vi "ActorPlugin-004-SpecificationCenter.vi"(0 "FTW Actor Instance Configuration":string="{\n  \"Identity\": \"ActorName\",\n  \"InboxAddress\": \"tcp://127.0.0.1:*\",\n  \"PublisherAddress\": \"tcp://127.0.0.1:*\",\n  \"DebugEnableInboxLogging\": false,\n  \"DebugEnableJobLogging\": false,\n  \"DebugShowPanel\": false\n}", 11 "Error In":errorcluster) -> (15 "Error":errorcluster)   [LabVIEW 2013, in "ERP-SpecificationManager.lvclass"]
uses:
  Actors/ERP-Specification Center/ERP-SpecificationManager.lvclass
  Actors/ERP-Specification Center/Controls/Spec-ManageExisting.ctl
  Actors/ERP-Specification Center/Controls/Spec-CreateNew.ctl
  Actors/ERP-Specification Center/ERP-SpecificationManager.lvclass/ERP-SpecificationManager.ctl
  ftw-dataflow/Actor/src/Instance/FTW-ActorInstance.lvclass
  ftw-dataflow/Actor/src/Message/Request/FTW-Message-IncomingRequest.lvclass
  ERP-ConfigPageNewFeather/PCert-ConfigPageNF.lvclass
panel:
  in  "Spec New":T1
  in  "Spec Manager":T2
  in  "Tab Control":T3(tab)
  in  "Refresh Table":bool
  in  "Delete Part":bool
  in  "Tables":u16(ring) items=["Aluminum Oxide Items", "CCW Items", "Other Items", "Probe Clean Items", "Probe Form Items", "Probe Lap Items", "Probe Polish Items", "Probe Scrub Items"]
  in  "Udpate Description":bool
  in  "Description Updater":string
  in  "Clear Search":bool
  in  "Part Number":string
  in  "Search Button":bool
  in  "Specification Table":string[][](table)
  # "Specification Controls"
  # "Welcome to the ITS Specification Manager\nPlease use the Controls below to \naccess the system."
  # "Update Part Number Description Option"
  # "Search Controls"
  # "Table Selection"
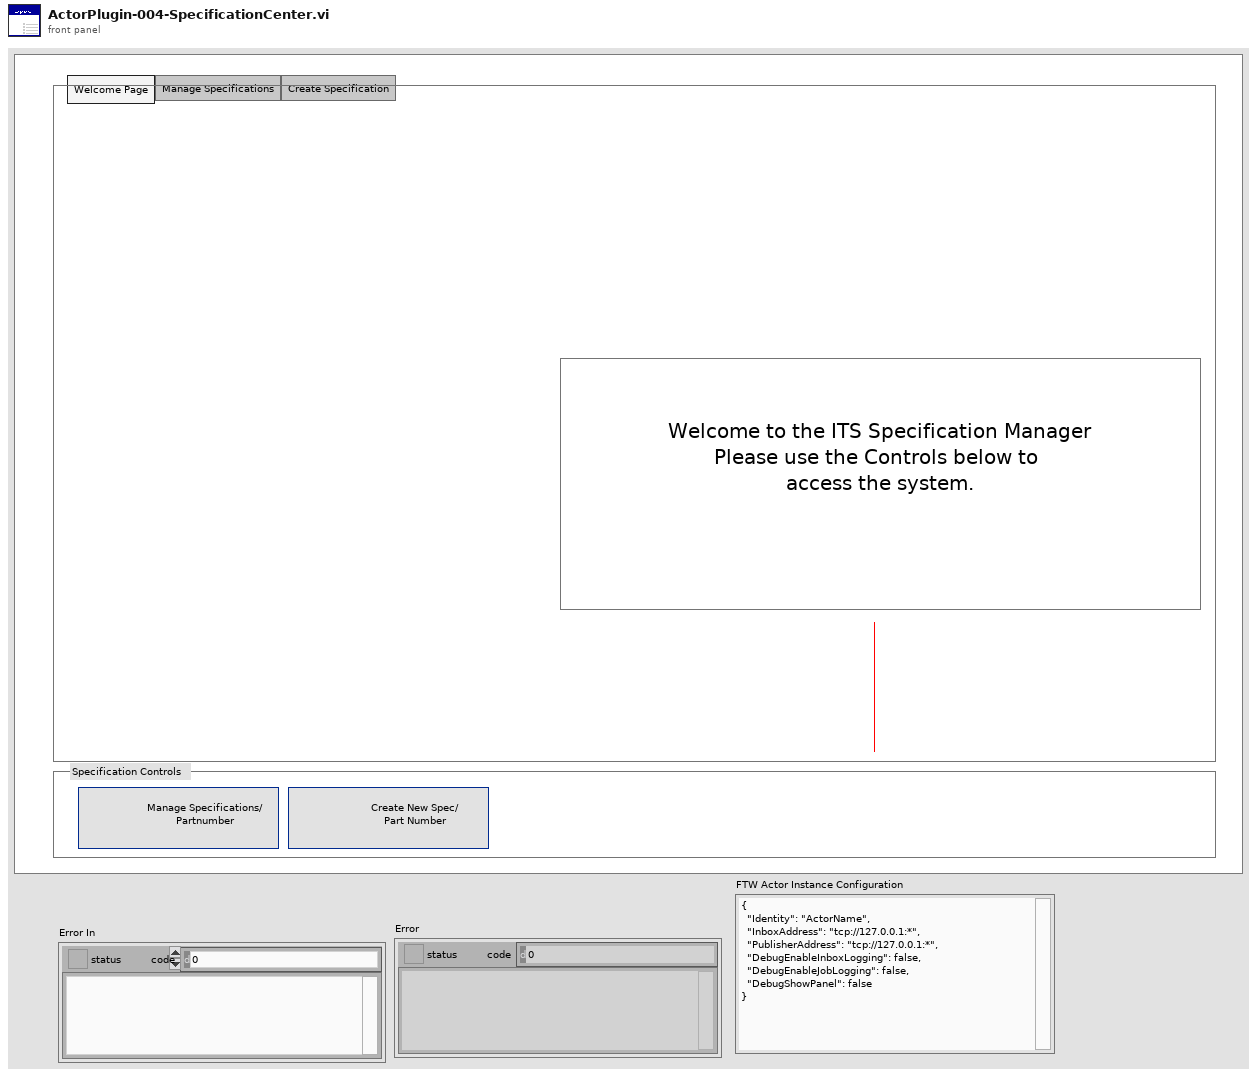
[diagram p1: front panel]
types:
  T1 = typedef "ERP-SpecificationManager.lvclass/Spec-CreateNew.ctl" = bool
  T2 = typedef "ERP-SpecificationManager.lvclass/Spec-ManageExisting.ctl" = bool
  T3 = enum32{"Welcome Page", "Manage Specifications", "Create Specification"}
  T4 = cluster{"Incoming Requests":refnum<event-registration>}
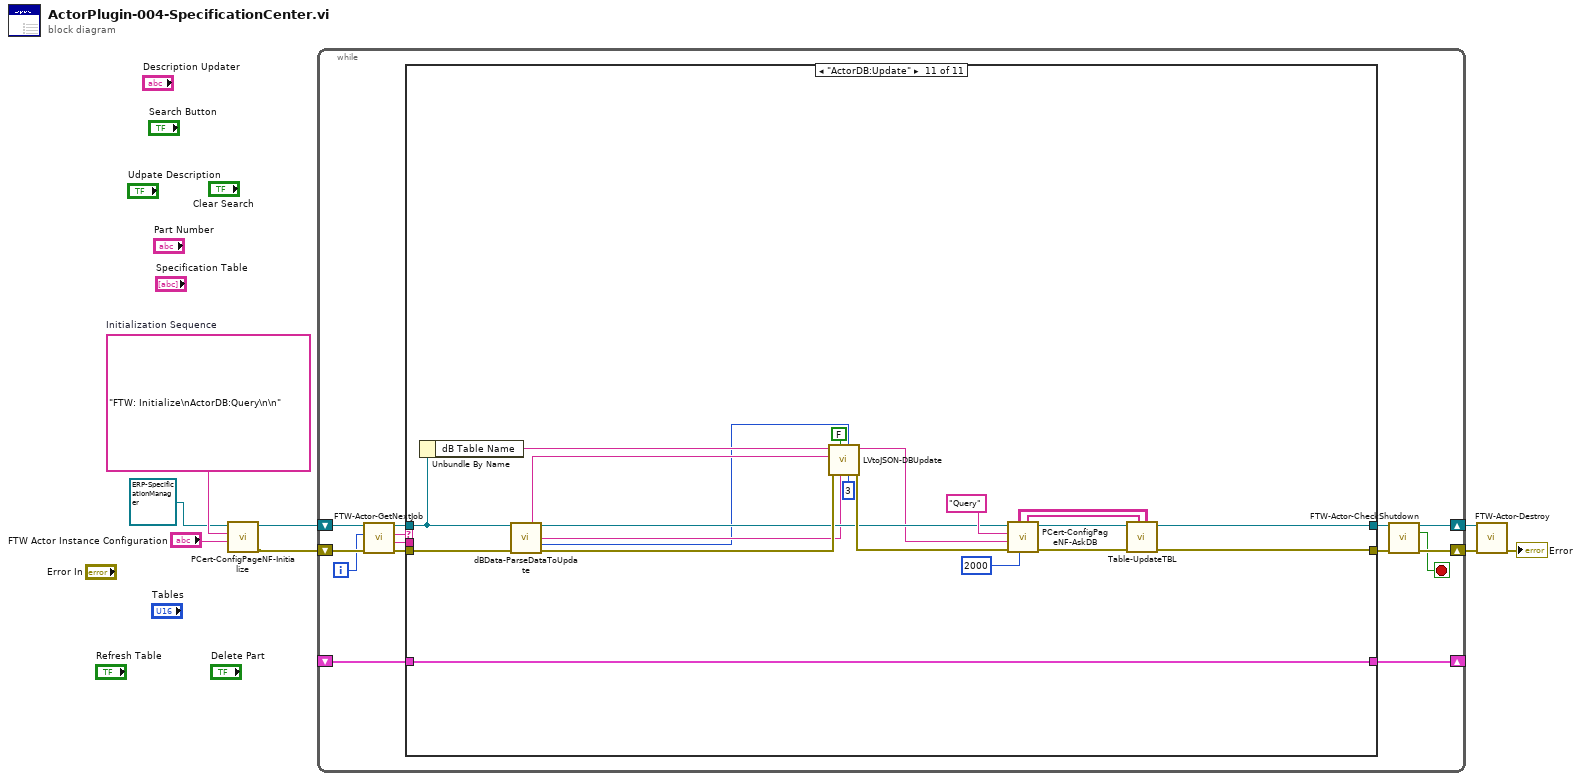
[diagram p0: block diagram]
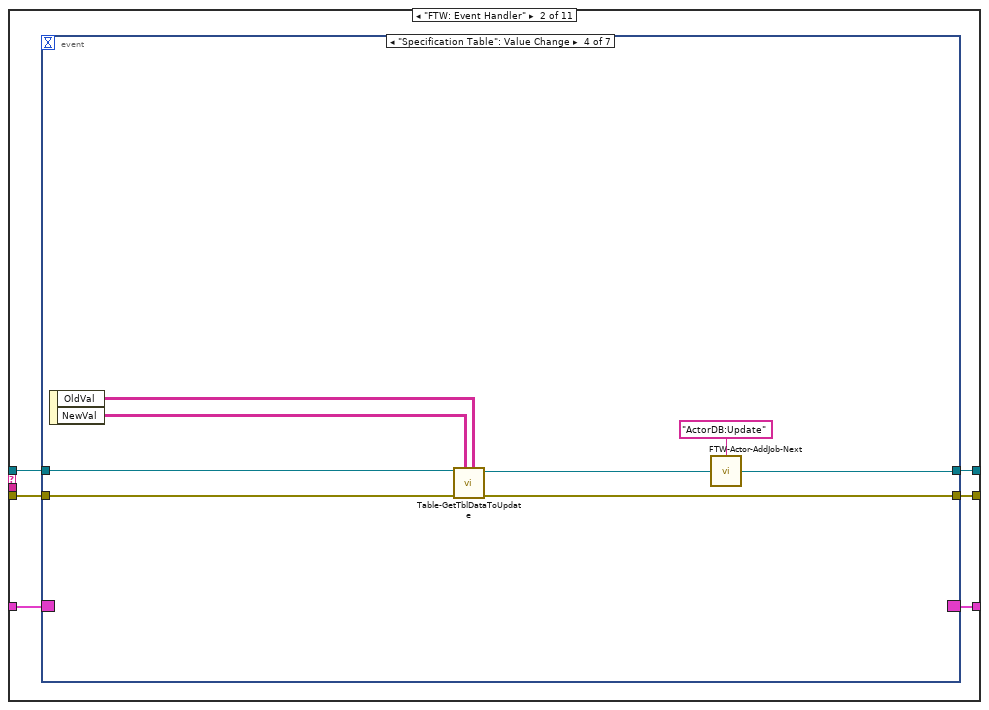
[diagram p3: hidden frame]
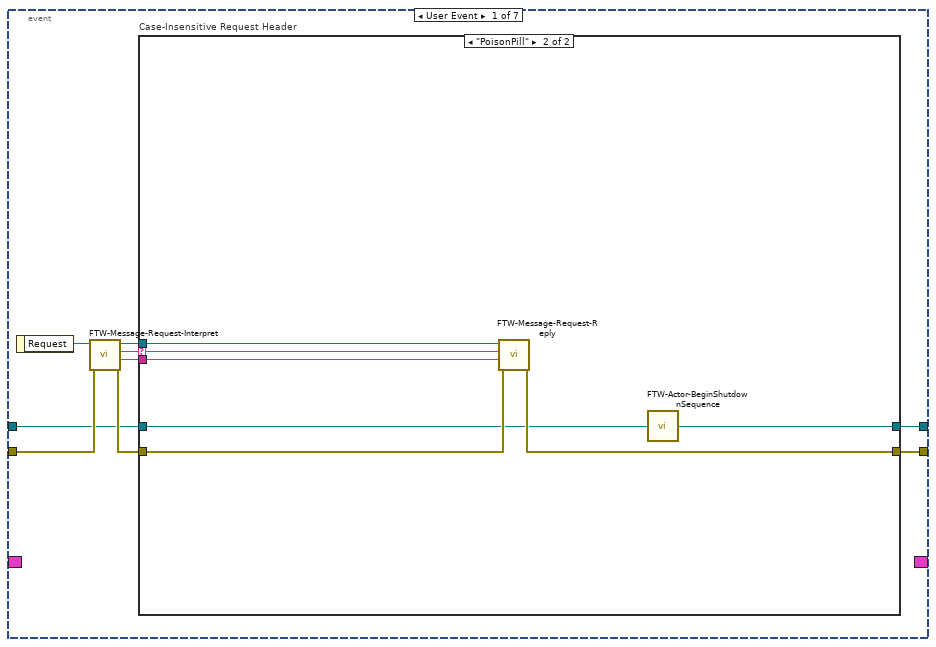
[diagram p4: hidden frame]
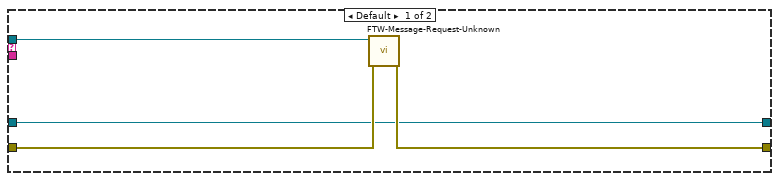
[diagram p5: hidden frame]
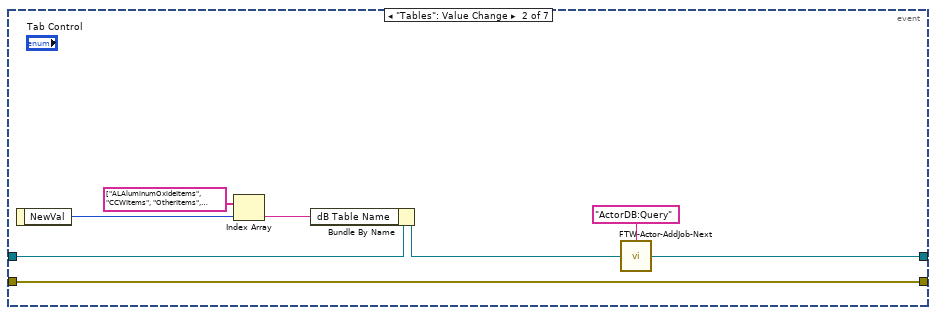
[diagram p6: hidden frame]
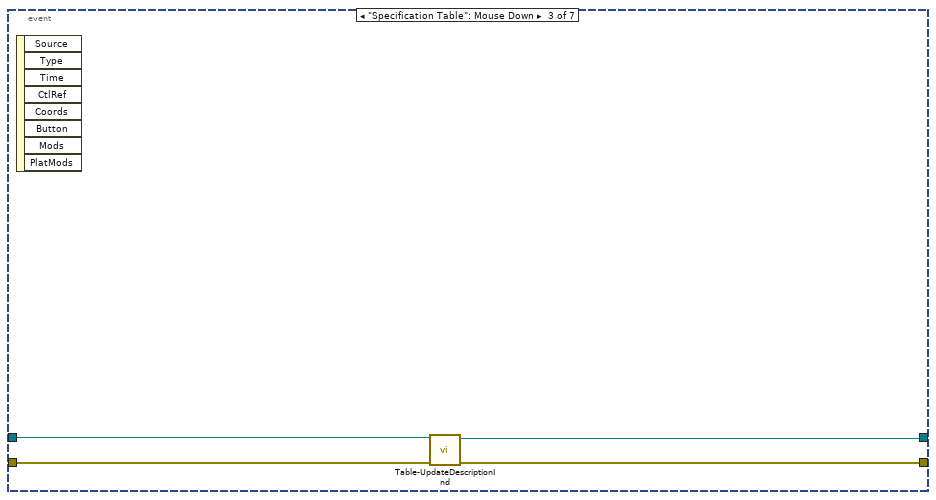
[diagram p7: hidden frame]
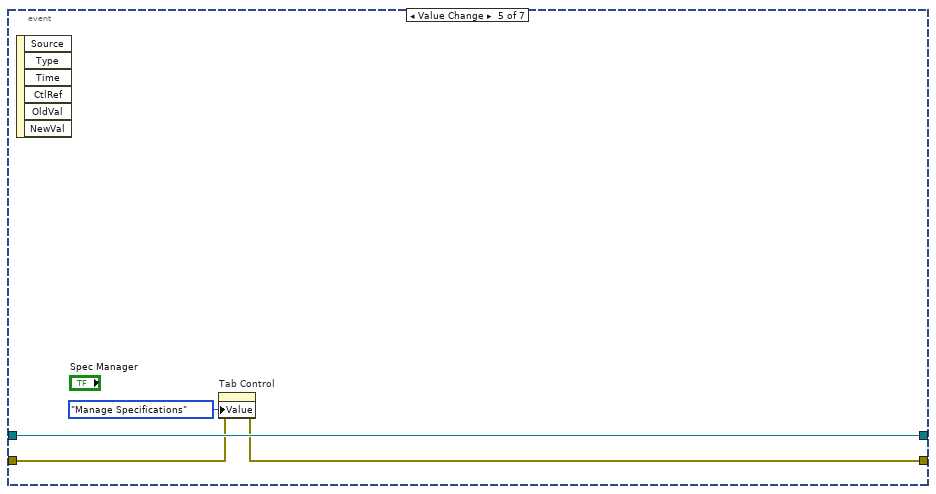
[diagram p8: hidden frame]
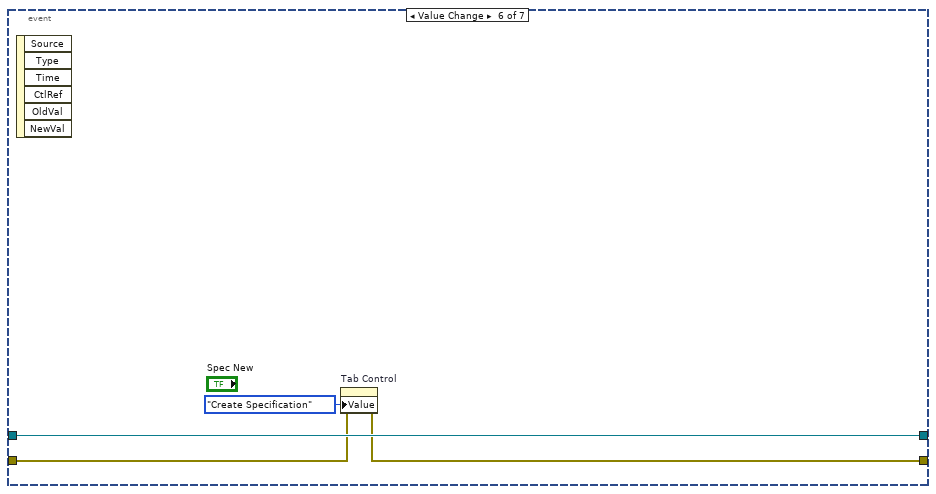
[diagram p9: hidden frame]
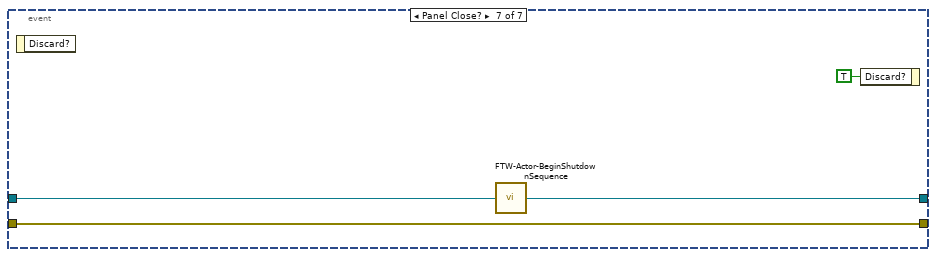
[diagram p10: hidden frame]
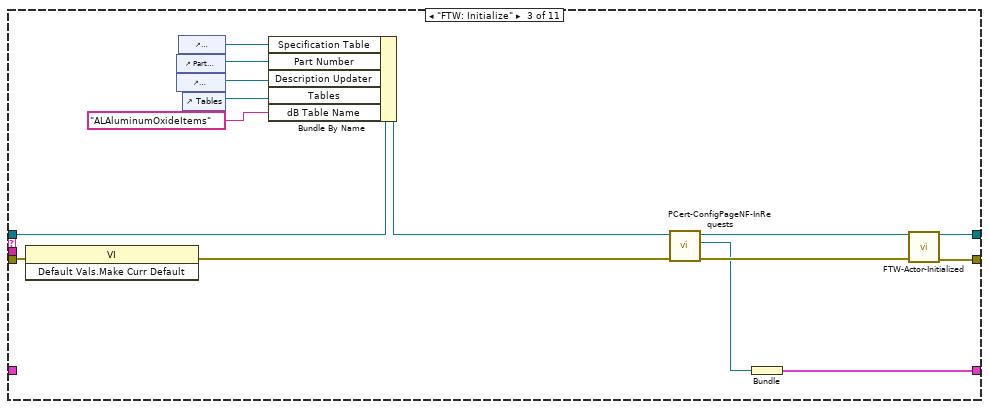
[diagram p11: hidden frame]
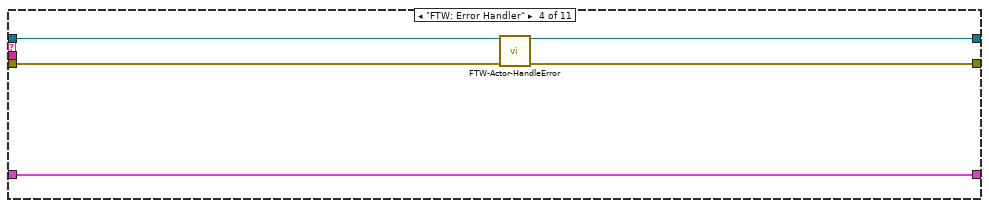
[diagram p12: hidden frame]
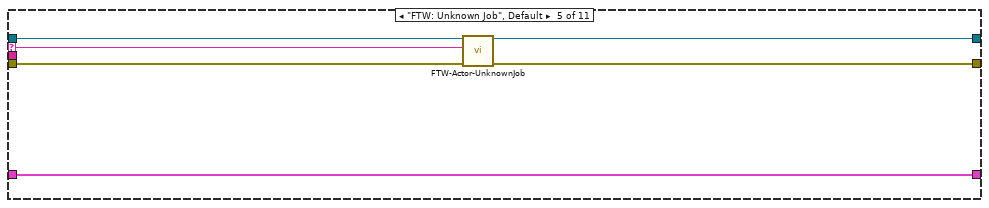
[diagram p13: hidden frame]
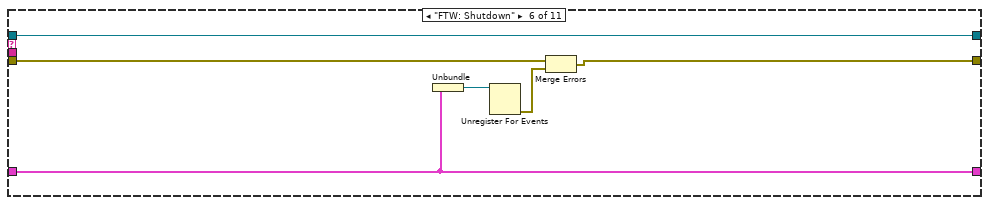
[diagram p14: hidden frame]
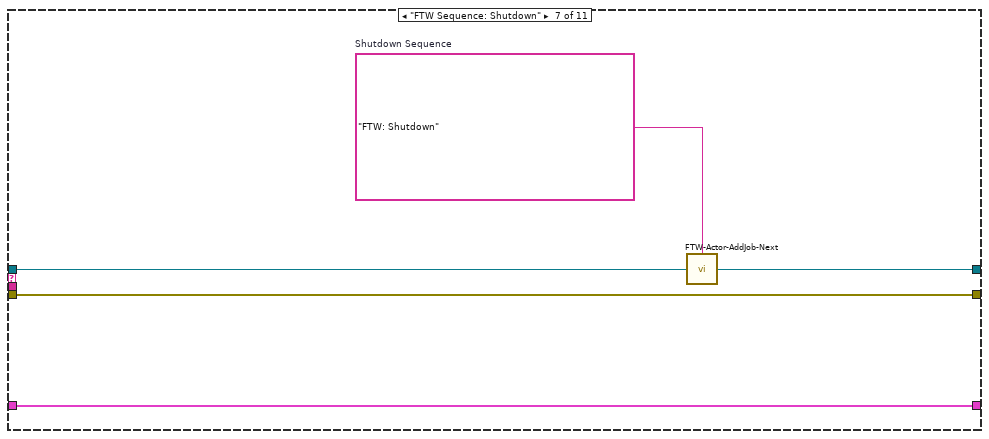
[diagram p15: hidden frame]
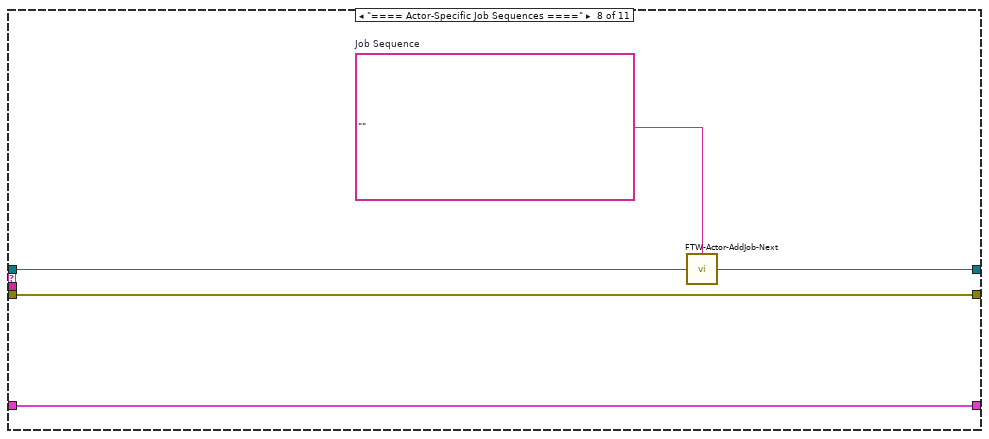
[diagram p16: hidden frame]
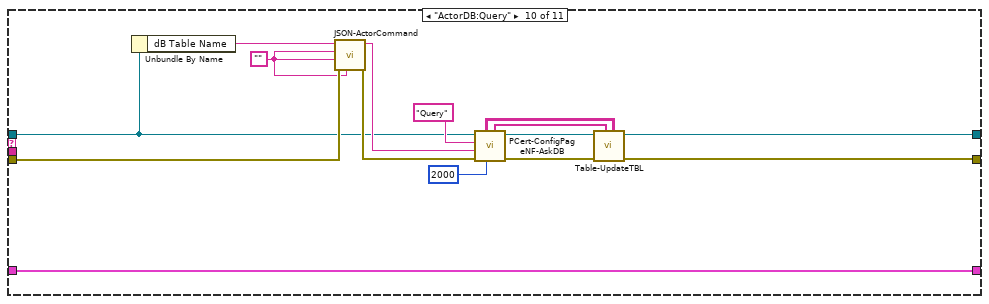
[diagram p18: hidden frame]
diagram:
  w5 = "FTW: Initialize\nActorDB:Query\n\n"  # Initialization Sequence
  n1 = call-dynamic "PCert-ConfigPageNF-Initialize.vi"("FTW Actor Instance Configuration"="FTW Actor Instance Configuration", "Initialization Job Sequence"=w5, "ERP-ConfigPageNF.lvclass"=refnum<class "ERP-SpecificationManager.lvclass"> refnum ("ERP-SpecificationManager.lvclass")) -> ("error out"=w3:errorcluster, "ERP-ConfigPageNF out"=w4:refnum<class "ERP-SpecificationManager.lvclass">)  [unwired: 7 in]
  n2 = while {
    shift-right: [w12] -> w7
    shift-left: w3 -> [w19]
    shift-right: [w9] -> _
    shift-left: _ -> [w22]
    shift-right: [w14] -> w8
    shift-left: w4 -> [w21]
    i -> [w10]
    stop <- w11 stop-if-true
    n3 = call "FTW-Actor-GetNextJob.vi"("error in"=w19, "Jobs Performed"=w10, "FTW Actor Instance"=w21) -> ("error out"=w18:errorcluster, "Job Data"=w16:string, "Job Name"=w17:string, "FTW Actor Instance out"=w20:refnum<class "ERP-SpecificationManager.lvclass">)  [unwired: 5 in]
    n4 = case shown="\"ActorDB:Update\"" w17 {
      selector: w17 -> [_ _ _ _ w104 _ _ _ _ _ _]
      tunnel: [w24 w31 w97 w99 w107 w113 w119 w124 w128 w134 w158] -> w13
      tunnel: w18 -> [w24 w30 w86 w101 w108 w110 w119 w124 w128 w138 w152]
      tunnel: w22 -> [w25 w26 _ w103 w109 w115 w120 w125 w127 w143 w164]
      tunnel: [w25 w29 w93 w103 w109 w115 w120 w125 w127 w143 w164] -> w9
      tunnel: w16 -> [_ _ _ _ _ _ _ _ _ _ _]
      tunnel: [w23 w28 w98 w100 w105 w111 w117 w122 w126 w136 w160] -> w15
      tunnel: w20 -> [w23 w27 w92 w102 w106 w111 w118 w123 w126 w131 w150]
      frame "==== Featherweight Framework Jobs ====" {
      }
      frame "FTW: Event Handler" {
        n5 = event shown="[3] \"Specification Table\": Value Change" {
          selector: w26 -> [_ _ _ _ _ _ _]
          dyn-events: [_ _ _ _ _ _ _] -> w29
          timeout: _ -> [_ _ _ _ _ _ _]
          tunnel: [w37 w59 w62 w67 w73 w76 w82] -> w31
          tunnel: w30 -> [w38 w59 w63 w69 w74 w77 w82]
          tunnel: [w36 w58 w60 w64 w75 w79 w80] -> w28
          tunnel: w27 -> [w35 w53 w61 w68 w75 w79 w81]
          event User Event {
            n6 = event-data() -> ("Request"=w39:refnum<class "FTW-Message-IncomingRequest.lvclass">)  [unwired: 1 in]
            n7 = call "FTW-Message-Request-Interpret.vi"("error in"=w38, "FTW Incoming Request"=w39) -> ("error out"=w40:errorcluster, "Request Body"=w33:string, "Request Header"=w34:string, "FTW Incoming Request out"=w32:refnum<class "FTW-Message-IncomingRequest.lvclass">)  [unwired: 6 in]
            n8 = case "Case-Insensitive Request Header" shown="\"PoisonPill\"" w34 {
              selector: w34 -> [_ w46]
              tunnel: [w43 w48] -> w37
              tunnel: w40 -> [w44 w49]
              tunnel: [w41 w51] -> w36
              tunnel: w35 -> [w41 w47]
              tunnel: w33 -> [_ w45]
              tunnel: w32 -> [w42 w50]
              frame Default {
                n9 = call "FTW-Message-Request-Unknown.vi"("error in"=w44, "FTW Incoming Request"=w42) -> ("error out"=w43:errorcluster)  [unwired: 9 in]
              }
              frame "PoisonPill" {
                n10 = call "FTW-Message-Request-Reply.vi"("error in"=w49, "Response Body"=w45, "Response Header"=w46, "FTW Incoming Request"=w50) -> ("error out"=w48:errorcluster)  [unwired: 6 in, 1 out]
                n11 = call "FTW-Actor-BeginShutdownSequence.vi"("FTW Actor Instance"=w47) -> ("FTW Actor Instance out"=w51:refnum<class "ERP-SpecificationManager.lvclass">)  [unwired: 3 in]
              }
            }
          }
          event "Tables": Value Change {
            n12 = event-data() -> ("NewVal"=w55:u16)  [unwired: 1 in]
            n13 = Index Array(array=string[] ["ALAluminumOxideItems", "CCWItems", "OtherItems", "ProbeCleanItems", "ProbeFormItems", "ProbeLapItems", "ProbePolishItems", "ProbeScrubItems"] ("Strings []"), index=w55) -> (element=w54:string)
            n14 = Bundle By Name(cluster=w53, "dB Table Name"=w54) -> (w52:refnum<class "ERP-SpecificationManager.lvclass">)
            n15 = call "FTW-Actor-AddJob-Next.vi"("Add Next in Job Queue"="ActorDB:Query", "FTW Actor Instance"=w52) -> ("FTW Actor Instance out"=w58:refnum<class "ERP-SpecificationManager.lvclass">)  [unwired: 2 in]
          }
          event "Specification Table": Mouse Down {
            n16 = event-data() -> ()  [unwired: 1 in, 8 out]
            n17 = call "Table-UpdateDescriptionInd.vi"("error in (no error)"=w63, "ERP-SpecificationManager in"=w61) -> ("error out"=w62:errorcluster, "ERP-SpecificationManager out"=w60:refnum<class "ERP-SpecificationManager.lvclass">)  [unwired: 8 in]
          }
          event "Specification Table": Value Change {
            n18 = event-data() -> ("OldVal"=w70:string[][], "NewVal"=w71:string[][])  [unwired: 1 in]
            n19 = call "Table-GetTblDataToUpdate.vi"("OldVal"=w70, "NewVal"=w71, "error in (no error)"=w69, "ERP-SpecificationManager in"=w68) -> ("error out"=w67:errorcluster, "ERP-SpecificationManager out"=w65:refnum<class "ERP-SpecificationManager.lvclass">)  [unwired: 6 in]
            n20 = call "FTW-Actor-AddJob-Next.vi"("Add Next in Job Queue"="ActorDB:Update", "FTW Actor Instance"=w65) -> ("FTW Actor Instance out"=w64:refnum<class "ERP-SpecificationManager.lvclass">)  [unwired: 2 in]
          }
          event Value Change {
            n21 = event-data() -> ()  [unwired: 1 in, 6 out]
            n22 = property on="Tab Control" class="TabCtl (strict)"(error in=w74, "Value"=T3."Manage Specifications" ("Tab Control")) -> (error out=w73:errorcluster)  [unwired: 1 in, 1 out]
          }
          event Value Change {
            n23 = event-data() -> ()  [unwired: 1 in, 6 out]
            n24 = property on="Tab Control" class="TabCtl (strict)"(error in=w77, "Value"=T3."Create Specification" ("Tab Control")) -> (error out=w76:errorcluster)  [unwired: 1 in, 1 out]
          }
          event Panel Close? {
            n25 = event-data() -> ()  [unwired: 1 in, 1 out]
            n26 = call "FTW-Actor-BeginShutdownSequence.vi"("FTW Actor Instance"=w81) -> ("FTW Actor Instance out"=w80:refnum<class "ERP-SpecificationManager.lvclass">)  [unwired: 3 in]
            n27 = event-data("Discard?"=TRUE) -> ()  [unwired: 1 in, 1 out]
          }
        }
      }
      frame "FTW: Initialize" {
        n28 = invoke class="VI" method="Default Vals.Make Curr Default"(error in=w86) -> (error out=w85:errorcluster)  [unwired: 2 in, 2 out]
        n29 = control-ref of="Part Number"() -> (w89:refnum<vi>)
        n30 = control-ref of="Description Updater"() -> (w88:refnum<vi>)
        n31 = control-ref of="Specification Table"() -> (w90:refnum<vi>)
        n32 = control-ref of="Tables"() -> (w87:refnum<vi>)
        n33 = Bundle By Name(cluster=w92, "Specification Table"=w90, "Part Number"=w89, "Description Updater"=w88, "Tables"=w87, "dB Table Name"="ALAluminumOxideItems") -> (w91:refnum<class "ERP-SpecificationManager.lvclass">)
        n34 = call "PCert-ConfigPageNF-InRequests.vi"("error in (no error)"=w85, "ERP-ConfigPageNF in"=w91) -> ("error out"=w95:errorcluster, "Incoming Requests"=w94:refnum<event-registration>, "ERP-ConfigPageNF out"=w96:refnum<class "ERP-SpecificationManager.lvclass">)  [unwired: 7 in]
        n35 = Bundle("Incoming Requests"=w94) -> (w93:T4)  [unwired: 1 in]
        n36 = call-dynamic "FTW-Actor-Initialized.vi"("FTW Actor Instance"=w96, "error in"=w95) -> ("FTW Actor Instance out"=w98:refnum<class "ERP-SpecificationManager.lvclass">, "error out"=w97:errorcluster)  [unwired: 12 in]
      }
      frame "FTW: Error Handler" {
        n37 = call-dynamic "FTW-Actor-HandleError.vi"("FTW Actor Instance"=w102, "error in"=w101) -> ("FTW Actor Instance out"=w100:refnum<class "ERP-SpecificationManager.lvclass">, "error out"=w99:errorcluster)  [unwired: 11 in, 1 out]
      }
      frame "FTW: Unknown Job", Default {
        n38 = call-dynamic "FTW-Actor-UnknownJob.vi"("FTW Actor Instance"=w106, "Unknown Job"=w104, "error in"=w108) -> ("FTW Actor Instance out"=w105:refnum<class "ERP-SpecificationManager.lvclass">, "error out"=w107:errorcluster)  [unwired: 11 in]
      }
      frame "FTW: Shutdown" {
        n39 = Unbundle(w115) -> ("Incoming Requests"=w114:refnum<event-registration>)
        n40 = Unregister For Events(event registration refnum=w114) -> (error out=w112:errorcluster)  [unwired: 1 in]
        n41 = Merge Errors(w110, w112) -> (w113:errorcluster)
      }
      frame "FTW Sequence: Shutdown" {
        w116 = "FTW: Shutdown"  # Shutdown Sequence
        n42 = call "FTW-Actor-AddJob-Next.vi"("Add Next in Job Queue"=w116, "FTW Actor Instance"=w118) -> ("FTW Actor Instance out"=w117:refnum<class "ERP-SpecificationManager.lvclass">)  [unwired: 2 in]
      }
      frame "==== Actor-Specific Job Sequences ====" {
        w121 = ""  # Job Sequence
        n43 = call "FTW-Actor-AddJob-Next.vi"("Add Next in Job Queue"=w121, "FTW Actor Instance"=w123) -> ("FTW Actor Instance out"=w122:refnum<class "ERP-SpecificationManager.lvclass">)  [unwired: 2 in]
      }
      frame "==== Actor-Specific Jobs ====" {
      }
      frame "ActorDB:Query" {
        w129 = ""
        n44 = Unbundle By Name(w131) -> ("dB Table Name"=w130:string)
        n45 = call "JSON-ActorCommand.vi"("Payload"=w129, "error in"=w138, "Reply Command"=w129, "SQL Statement"=w129, "Table"=w130) -> ("error out"=w141:errorcluster, "Output JSON Object"=w142:string)  [unwired: 5 in]
        n46 = call "PCert-ConfigPageNF-AskDB.vi"("Timeout"=2000, "error in (no error)"=w141, "Request Body"=w142, "Request Header"="Query" ("Message Header"), "ERP-ConfigPageNF in"=w131) -> ("error out"=w135:errorcluster, "ERP-ConfigPageNF out"=w137:refnum<class "ERP-SpecificationManager.lvclass">, "Raw Column Data From DB"=w133:string[], "Raw Data From DB"=w132:string[][])  [unwired: 2 in, 1 out]
        n47 = call "Table-UpdateTBL.vi"("Data for Front Panel Table"=w132, "Column Headers"=w133, "error in (no error)"=w135, "ERP-SpecificationManager in"=w137) -> ("error out"=w134:errorcluster, "ERP-SpecificationManager out"=w136:refnum<class "ERP-SpecificationManager.lvclass">)  [unwired: 6 in]
      }
      frame "ActorDB:Update" {
        n48 = Unbundle By Name(w150) -> ("dB Table Name"=w153:string)
        n49 = call "dBData-ParseDataToUpdate.vi"("ERP-SpecificationManager in"=w150, "error in (no error)"=w152) -> ("SQL Statement"=w148:string, "ERP-SpecificationManager out"=w149:refnum<class "ERP-SpecificationManager.lvclass">, "Payload"=w147:string, "Column"=w145:i32, "error out"=w151:errorcluster)  [unwired: 9 in]
        n50 = call "LVtoJSON-DBUpdate.vi"("Datatype"=3 ("Column Number"), "Column Number"=w145, "Payload"=w147, "Update All"=FALSE, "error in"=w151, "SQL Statement"=w148, "Table"=w153) -> ("error out"=w154:errorcluster, "Output JSON Object"=w146:string)  [unwired: 3 in]
        n51 = call "PCert-ConfigPageNF-AskDB.vi"("Timeout"=2000, "error in (no error)"=w154, "Request Body"=w146, "Request Header"="Query" ("Message Header"), "ERP-ConfigPageNF in"=w149) -> ("error out"=w159:errorcluster, "ERP-ConfigPageNF out"=w161:refnum<class "ERP-SpecificationManager.lvclass">, "Raw Column Data From DB"=w157:string[], "Raw Data From DB"=w156:string[][])  [unwired: 2 in, 1 out]
        n52 = call "Table-UpdateTBL.vi"("Data for Front Panel Table"=w156, "Column Headers"=w157, "error in (no error)"=w159, "ERP-SpecificationManager in"=w161) -> ("error out"=w158:errorcluster, "ERP-SpecificationManager out"=w160:refnum<class "ERP-SpecificationManager.lvclass">)  [unwired: 6 in]
      }
    }
    n53 = call "FTW-Actor-CheckShutdown.vi"("FTW Actor Instance"=w15, "error in"=w13) -> ("FTW Actor Instance out"=w14:refnum<class "ERP-SpecificationManager.lvclass">, "Shutdown?"=w11:bool, "error out"=w12:errorcluster)  [unwired: 11 in]
  }
  n54 = call-dynamic "FTW-Actor-Destroy.vi"("FTW Actor Instance"=w8, "error in"=w7) -> ("error out"=→"Error":errorcluster)  [unwired: 13 in]
